vi "Get Position with Compas.vi"(9 "Heading (deg)":dbl, 10 "Delta y":i16, 11 "Delta x":i16) -> (2 "y out":dbl, 3 "x out":dbl)   [LabVIEW 2012]
uses:
  <vilib>/Analysis/coordinate.llb/2D Cartesian Coordinate Rotation (Scalar).vi
  <vilib>/Analysis/NI_AALPro.lvlib
panel:
  in  "CPI scale":sgl=70866.0
  # "Meters: 70866\ncm: 708.66"
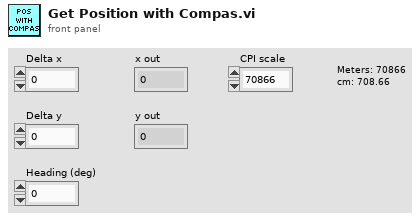
[diagram p1: front panel]
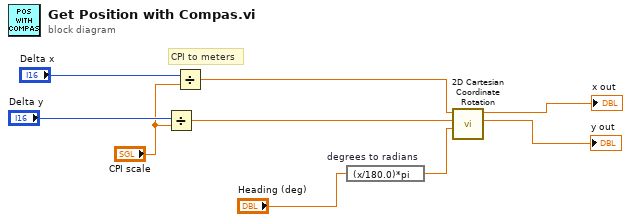
[diagram p0: block diagram]
diagram:
  # "CPI to meters"
  n1 = Divide(x="Delta y", y="CPI scale") -> (x/y=w5:sgl)
  n2 = Divide(x="Delta x", y="CPI scale") -> (x/y=w4:sgl)
  n3 = expression code="(x/180.0)*pi" "degrees to radians"("Heading (deg)") -> (w3:dbl)
  n4 = call-poly <vilib>:"2D Cartesian Coordinate Rotation.vi"("theta"=w3, "y"=w5, "x"=w4) -> ("y out"=→"y out":dbl, "x out"=→"x out":dbl)  [unwired: 6 in, 1 out]
